vi "EditVariant.vi"(8 "Error":errorcluster, 9 "Variant":variant, 10 "Tag":string, 11 "Tree in":refnum<class "Tree.lvclass">) -> (0 "Error":errorcluster, 1 "ItemData":T1, 2 "Found?":bool, 3 "Tree out":refnum<class "Tree.lvclass">)   [LabVIEW 2021, in "Tree.lvlib" / "Tree.lvclass"]
uses:
  Tree.lvclass
  Private/TreeControllerTag.ctl
  Tree.lvclass/Tree.ctl
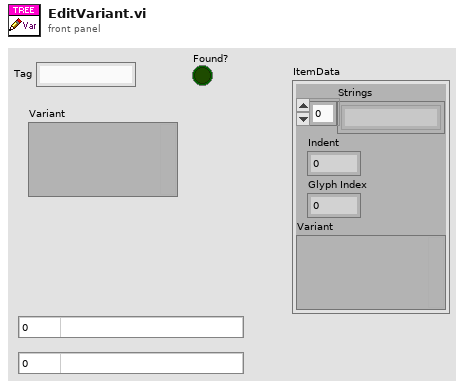
[diagram p1: front panel]
types:
  T1 = cluster{"Strings":string[], "Indent":i32, "Glyph Index":i32, "Variant":variant}
  T2 = cluster{enum16{"EditStrings", "EditGraph", "EditVariant"}, "Tag":string, "Value":variant}
  T3 = enum16{"EditStrings", "EditGraph", "EditVariant"}
  T4 = cluster{"Found":bool, "ItemData":cluster{"Strings":string[], "Indent":i32, "Glyph Index":i32, "Variant":variant}}
  T5 = typedef "Tree.lvlib/Tree.lvclass/TreeControllerTag.ctl" = enum8{"Null", "1. Add item", "2. Delete item", "3. Get All Tree Data", "4. Drag Starting", "5. Drag Ended", "6. Add Tree Values", "7. Get Item Value", "8. Edit Item", "9. StepBack", "10. Filter"}
  T6 = cluster{"cluster":cluster{enum16{"EditStrings", "EditGraph", "EditVariant"}, "Tag":string, "Value":variant}, "queue out":refnum<queue>}
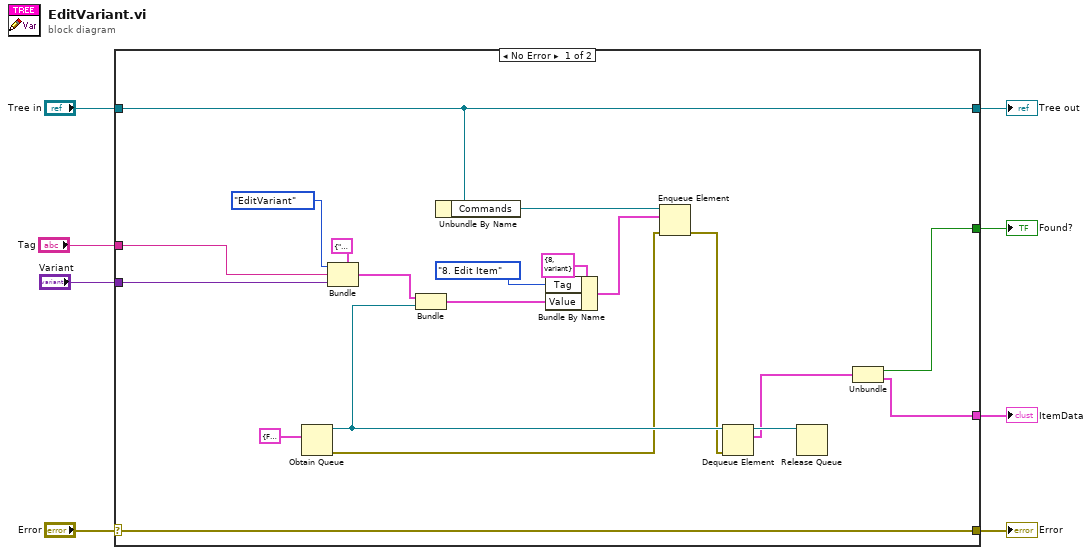
[diagram p0: block diagram]
diagram:
  n1 = case shown="No Error" "Error" {
    selector: "Error" -> [w28 w30]
    tunnel: [w28 w30] -> w7
    tunnel: [w27 w29] -> w5
    tunnel: "Tree in" -> [w27 w29]
    tunnel: "Variant" -> [w9 _]
    tunnel: [w15 _] -> w3
    tunnel: "Tag" -> [w19 _]
    tunnel: [w14 _] -> w1
    frame No Error {
      n2 = Obtain Queue(element data type=T4 {"Found"=FALSE, "ItemData"={"Strings"=[], "Indent"=0, "Glyph Index"=0, "Variant"=variant}} ("output cluster")) -> (queue out=w22:refnum<queue>, error out=w12:errorcluster)  [unwired: 4 in, 1 out]
      n3 = Bundle(cluster=T2 {enum."EditStrings", "Tag"="", "Value"=variant}, T3."EditVariant", "Tag"=w19, "Value"=w9) -> (w20:T2)
      n4 = Bundle("cluster"=w20, "queue out"=w22) -> (w23:T6)  [unwired: 1 in]
      n5 = Unbundle By Name(w27) -> ("Commands"=w26:refnum<queue>)
      n6 = Bundle By Name(cluster=cluster{"Tag":u8, "Value":variant} {"Tag"=8, "Value"=variant} ("element"), "Tag"=TreeControllerTag."8. Edit Item", "Value"=w23) -> (w24:cluster{"Tag":u8, "Value":variant})
      n7 = Enqueue Element(queue=w26, element=w24, error in (no error)=w12) -> (error out=w13:errorcluster)  [unwired: 1 in, 2 out]
      n8 = Dequeue Element(queue=w22, error in (no error)=w13) -> (queue out=w21:refnum<queue>, element=w16:T4)  [unwired: 1 in, 2 out]
      n9 = Release Queue(queue=w21) -> ()  [unwired: 2 in, 3 out]
      n10 = Unbundle(w16) -> ("Found"=w15:bool, "ItemData"=w14:T1)
    }
    frame Error {
    }
  }
  "Error" <- w7
  "Tree out" <- w5
  "Found?" <- w3
  "ItemData" <- w1
